vi "DAQmx.Create AO Tasks.vi"(8 "error in (no error)":errorcluster, 11 "DAQmx in":refnum<class "DAQmx.lvclass">) -> (0 "error out":errorcluster, 3 "DAQmx out":refnum<class "DAQmx.lvclass">)   [LabVIEW 2019, in "DAQmx.lvclass"]
uses:
  DAQmx.lvclass
  typedefs/DAQ.Config.AO--Cluster--Array.ctl
  typedefs/DAQ.Config.AO--Cluster.ctl
  typedefs/DAQ.Config.AO.Range--enum.ctl
  typedefs/DAQ.Config.Device Type--enum.ctl
  DAQmx.lvclass/DAQmx.ctl
  <vilib>/DAQmx/create/channels.llb/DAQmx Create Channel (AO-Voltage-Basic).vi
  <resource>/objmgr/daqmx.rc
panel:
  out "AO":T1 {"output terminal configuration" items=[""=-1, "Differential"=10106, "Pseudodifferential"=12529]}
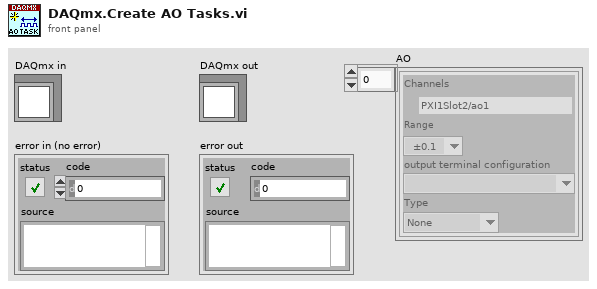
[diagram p1: front panel]
types:
  T1 = typedef "DAQmx.lvclass/DAQ.Config.AO--Cluster--Array.ctl" = T2[]
  T2 = typedef "DAQmx.lvclass/DAQ.Config.AO--Cluster.ctl" = cluster{"Channels":tag, "Range":T3, "output terminal configuration":i32, "Type":T4}
  T3 = typedef "DAQmx.lvclass/DAQ.Config.AO.Range--enum.ctl" = enum16{"±0.1", "±1.0", "±3.5", "±10.0", ""}
  T4 = typedef "DAQmx.lvclass/DAQ.Config.Device Type--enum.ctl" = enum16{"None", "USB-4431", "PXI-446x"}
  T5 = typedef "DAQmx.lvclass/DAQmx.Channel Map--Cluster.ctl" = cluster{"task":refnum<k21>, "Device":tag, "Offset":u32, "Count":u32}
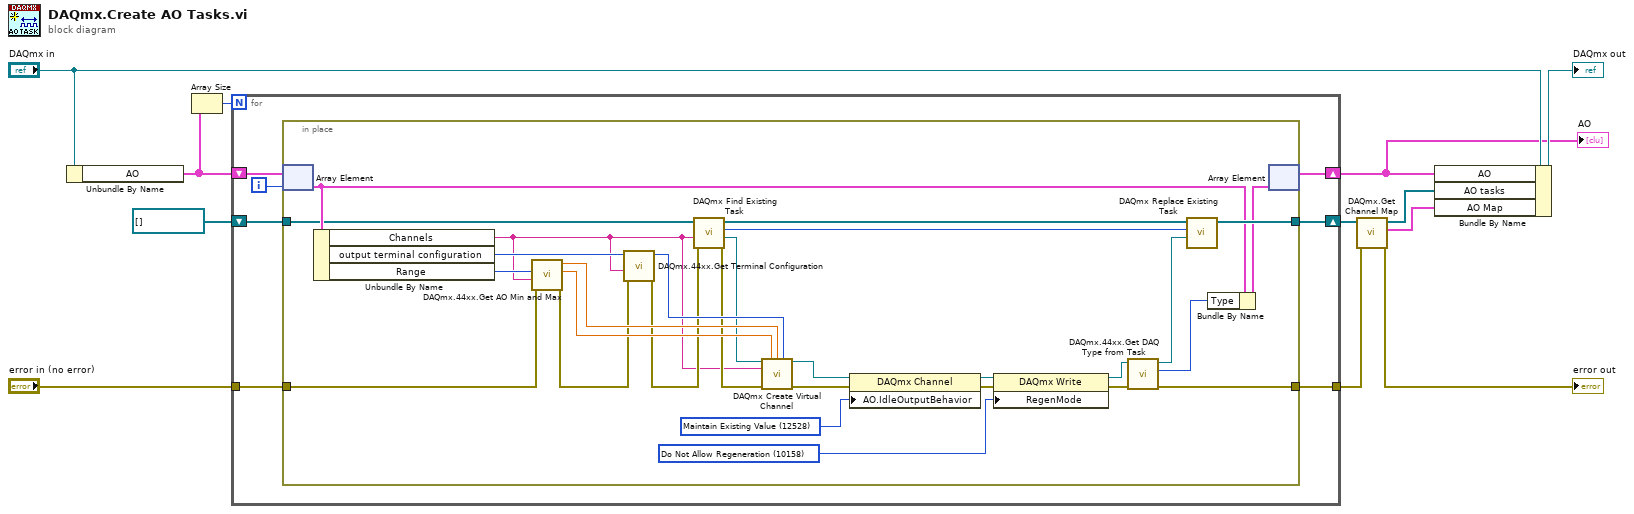
[diagram p0: block diagram]
diagram:
  n1 = Unbundle By Name("DAQmx in") -> ("AO"=w7:T1)
  n2 = Array Size(array=w7) -> (size(s)=w8:i32)
  n3 = for {
    N: w8 -> [_]
    tunnel: "error in (no error)" -> [w19]
    tunnel: [w18] -> w6
    shift-right: [w17] -> w3
    shift-left: refnum<k21>[] [] -> [w16]
    shift-right: [w14] -> w1
    shift-left: w7 -> [w15]
    i -> [w13]
    n4 = in-place {
      in-place-border: w19 -> [w47]
      in-place-border: [w45] -> w18
      in-place-border: [w37] -> w17
      in-place-border: w16 -> [w22]
      w41 = 10158 items=["Allow Regeneration"=10097, "Do Not Allow Regeneration"=10158] ("RegenMode")
      w40 = 12528 items=["Zero Volts"=12526, "High-Impedance"=12527, "Maintain Existing Value"=12528] ("AO.IdleOutputBehavior")
      n5 = in-place-array #1(w15, w13) -> (w25:T2)
      n6 = Unbundle By Name(w25) -> ("Channels"=w21:tag, "output terminal configuration"=w26:i32, "Range"=w24:T3)
      n7 = call "DAQmx.44xx.Get AO Min and Max.vi"("error in (no error)"=w47, "AO.channels"=w21, "AO.Range"=w24) -> ("error out"=w30:errorcluster, "AO.max"=w32:dbl, "AO.min"=w31:dbl)  [unwired: 6 in]
      n8 = call "DAQmx.44xx.Get Terminal Configuration.vi"("error in (no error)"=w30, "Channel in"=w21, "terminal configuration in"=w26) -> ("error out"=w29:errorcluster, "terminal configuration out"=w33:i32)  [unwired: 7 in]
      n9 = call "DAQmx Find Existing Task.vi"("error in (no error)"=w29, "Channels"=w21, "Tasks in"=w22) -> ("error out"=w28:errorcluster, "Task out"=w20:refnum<k21>, "Task Index"=w27:i32, "Tasks out"=w23:refnum<k21>[])  [unwired: 5 in]
      n10 = call-poly <vilib>:"DAQmx Create Virtual Channel.vi"("task in"=w20, "maximum value"=w32, "minimum value"=w31, "output terminal configuration"=w33, "physical channels"=w21, "error in"=w28) -> ("task out"=w39:refnum<k21>, "error out"=w44:errorcluster)  [unwired: 8 in]
      n11 = property class="DAQmx Channel"(reference=w39, error in=w44, "AO.IdleOutputBehavior"=w40) -> (reference out=w43:refnum<k21>, error out=w42:errorcluster)
      n12 = property class="DAQmx Write"(reference=w43, error in=w42, "RegenMode"=w41) -> (reference out=w38:refnum<k21>, error out=w46:errorcluster)
      n13 = call "DAQmx.44xx.Get DAQ Type from Task.vi"("error in (no error)"=w46, "Task in"=w38) -> ("error out"=w45:errorcluster, "DAQ Type"=w35:T4, "Task out"=w36:refnum<k21>)  [unwired: 5 in, 2 out]
      n14 = call "DAQmx Replace Existing Task.vi"("Task in"=w36, "Task Index"=w27, "Tasks in"=w23) -> ("Tasks out"=w37:refnum<k21>[])  [unwired: 8 in]
      n15 = Bundle By Name(cluster=w25, "Type"=w35) -> (w34:T2)
      n16 = in-place-array #1(w34) -> (w14:T1)  [unwired: 1 out]
    }
  }
  "AO" <- w1
  n17 = call "DAQmx.Get Channel Map.vi"("error in (no error)"=w6, "tasks in"=w3) -> ("error out"=→"error out":errorcluster, "Channel Map"=w4:T5[], "tasks out"=w2:refnum<k21>[])  [unwired: 7 in]
  n18 = Bundle By Name(cluster="DAQmx in", "AO"=w1, "AO tasks"=w2, "AO Map"=w4) -> (→"DAQmx out":refnum<class "DAQmx.lvclass">)
